vi "HEWH RLT Find TC Channel.vi"(7 "Program Channel Locations In":string[](array[string]), 8 "Error In":errorcluster, 9 "TC Data":string[][](array[string]), 11 "Station A Channels, MW100":string[][](array[string])=[["T1 - IN", "11"], ["T1 - OUT", "13"]]) -> (0 "Error Out":errorcluster, 3 "TC Data":string[][](array[string]))   [LabVIEW 2019]
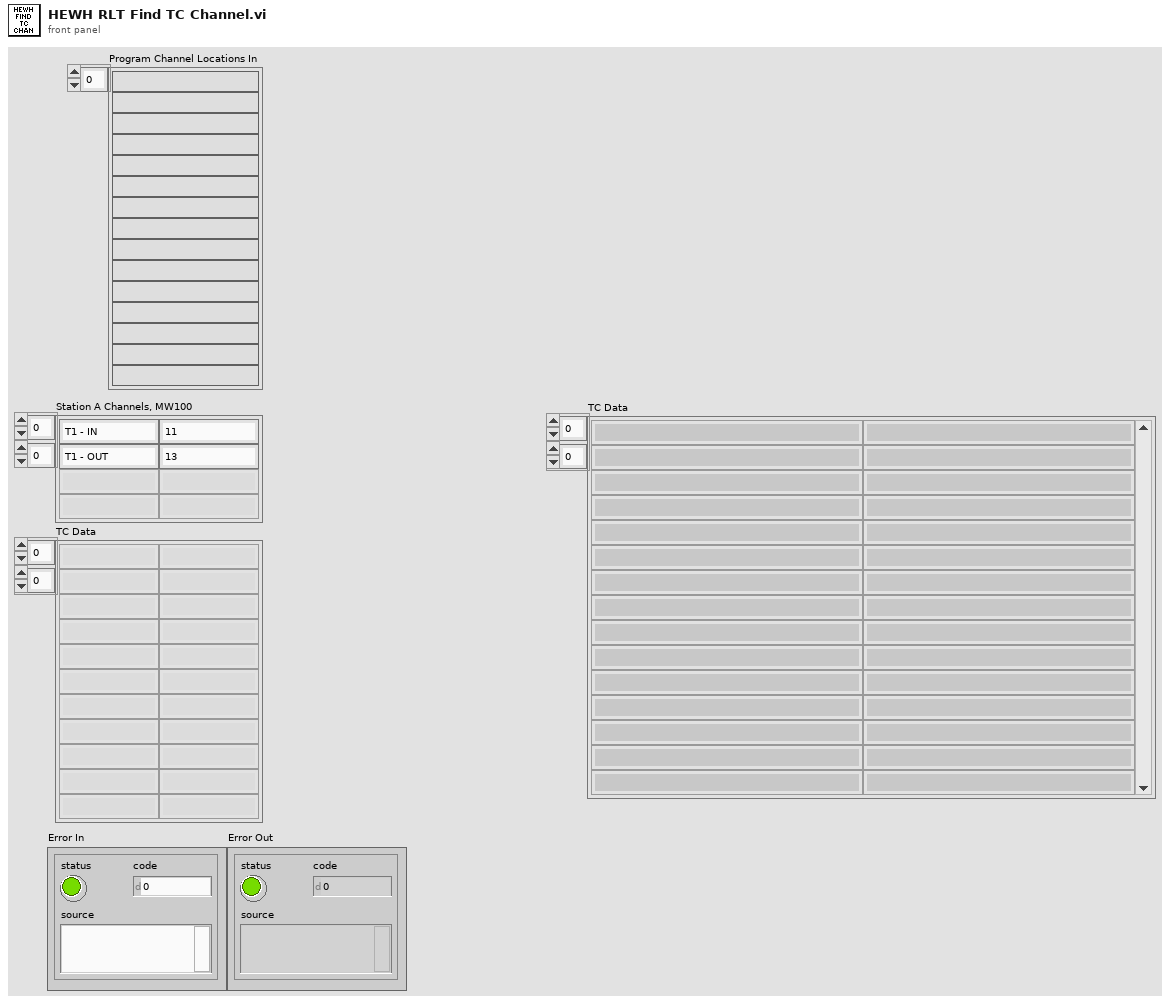
[diagram p1: front panel]
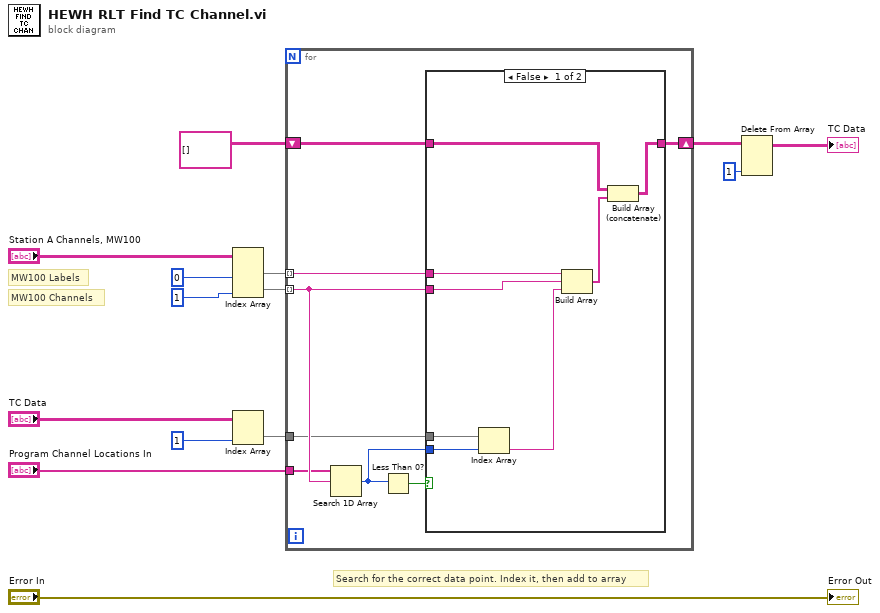
[diagram p0: block diagram]
diagram:
  # "MW100 Channels"
  # "MW100 Labels"
  # "Search for the correct data point. Index it, then add to array"
  n1 = Index Array(array="Station A Channels, MW100", index (col) #1=0 ("disabled index (col)"), index (col) #2=1 ("disabled index (col)")) -> (element #1=w2:string[], element #2=w3:string[])  [unwired: 2 in]
  n2 = Index Array(array="TC Data", index (col)=1 ("disabled index (col)")) -> (element=w7:string[])  [unwired: 1 in]
  n3 = for {
    tunnel: w3 -> [w17] mode=indexing
    shift-right: [w19] -> w14
    shift-left: string[][] [] -> [w20]
    tunnel: w2 -> [w18] mode=indexing
    tunnel: w7 -> [w16]
    tunnel: "Program Channel Locations In" -> [w15]
    n4 = Search 1D Array(1D array=w15, element=w17) -> (index of element=w22:i32)  [unwired: 1 in]
    n5 = Less Than 0?(x=w22) -> (x < 0?=w21:bool)
    n6 = case shown="False" w21 {
      tunnel: w22 -> [w30 _]
      tunnel: w20 -> [w26 w31]
      tunnel: [w24 w31] -> w19
      tunnel: w18 -> [w29 _]
      tunnel: w17 -> [w28 _]
      tunnel: w16 -> [w23 _]
      frame False {
        n7 = Index Array(array=w23, index=w30) -> (element=w27:string)
        n8 = Build Array(w29, w28, w27) -> (w25:string[])
        n9 = Build Array (concatenate)(w26, w25) -> (w24:string[][])
      }
      frame True {
      }
    }
  }
  n10 = Delete From Array(array=w14, index (col)=1 ("disabled index (col)")) -> (array with subset deleted=→"TC Data":string[][])  [unwired: 2 in, 1 out]
  "Error Out" <- "Error In"
